vi "parse_point32.vi"(4 "error in":errorcluster, 7 "msg in":string) -> (0 "error out":errorcluster, 2 "Point32":cluster{"x":sgl, "y":sgl, "z":sgl}, 3 "msg out":string)   [LabVIEW 2012]
doc: "Parses a message into pt 32"
uses:
  <userlib>/ROSforLV/ROS/parsing/std_msgs/subs/parse_float32_scalar.vi
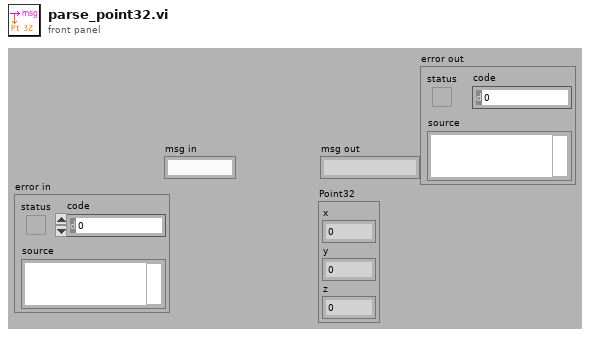
[diagram p1: front panel]
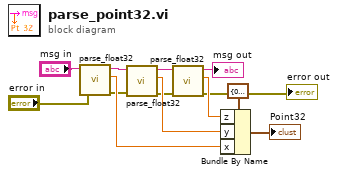
[diagram p0: block diagram]
diagram:
  n1 = call-poly <userlib>:"parse_float32.vi"("error in"="error in", "msg in"="msg in") -> ("error out"=w2:errorcluster, "number"=w5:sgl, "msg out"=w13:string)  [unwired: 3 in]
  n2 = call-poly <userlib>:"parse_float32.vi"("error in"=w2, "msg in"=w13) -> ("error out"=w1:errorcluster, "number"=w6:sgl, "msg out"=w12:string)  [unwired: 3 in]
  n3 = call-poly <userlib>:"parse_float32.vi"("error in"=w1, "msg in"=w12) -> ("error out"=→"error out":errorcluster, "number"=w7:sgl, "msg out"=→"msg out":string)  [unwired: 3 in]
  n4 = Bundle By Name(cluster=cluster{"x":sgl, "y":sgl, "z":sgl} {"x"=0.0, "y"=0.0, "z"=0.0} ("Point32"), "z"=w7, "y"=w6, "x"=w5) -> (→"Point32":cluster{"x":sgl, "y":sgl, "z":sgl})
